vi "Add Library.vi"(6 "Library Path":path, 8 "error in":errorcluster, 9 "Name Library":string, 10 "Project:Active Project":refnum<vi>) -> (0 "error out":errorcluster)   [LabVIEW 2021, in "_Template.lvlib" / "Script Strategy.lvlib"]
uses:
  Script Strategy.lvlib
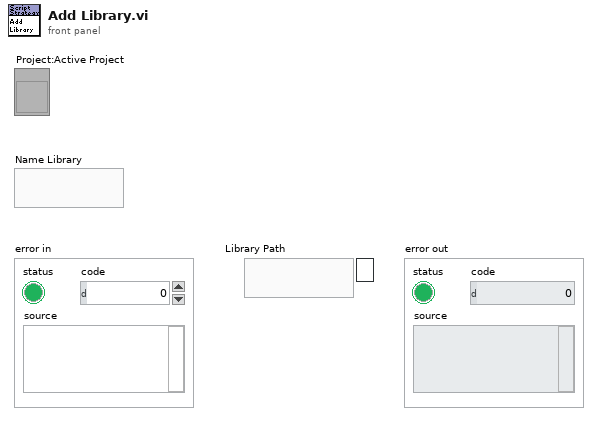
[diagram p1: front panel]
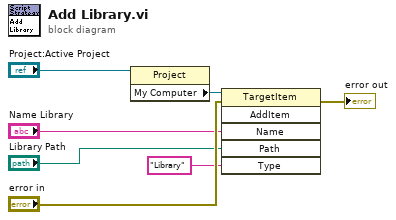
[diagram p0: block diagram]
diagram:
  n1 = property class="Project"(reference="Project:Active Project") -> ("My Computer"=w6:refnum<vi>)  [unwired: 1 in, 2 out]
  n2 = invoke class="TargetItem" method="AddItem"(reference=w6, error in="error in", "Name"="Name Library", "Path"="Library Path", "Type"="Library") -> (error out=→"error out":errorcluster)  [unwired: 1 in, 5 out]
